vi "ShuntConvert.vi"(1 "Potential drop":dbl) -> (0 "Current":dbl)   [LabVIEW 2013]
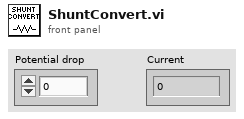
[diagram p1: front panel]
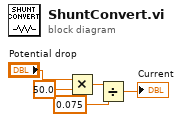
[diagram p0: block diagram]
diagram:
  n1 = Multiply(x="Potential drop", y=50.0) -> (x*y=w3:dbl)
  n2 = Divide(x=w3, y=0.075) -> (x/y=→"Current":dbl)
